vi "Get Children.vi"(8 "error in (no error)":errorcluster, 11 "Tag_LVOOP in":refnum<class "Tree Tag Class.lvclass">) -> (0 "error out":errorcluster, 1 "Child found?":bool, 2 "Children Tag Strings":string[](array[string]), 3 "Tag_LVOOP out":refnum<class "Tree Tag Class.lvclass">)   [LabVIEW 2012, in "Tree Tools.lvlib" / "Tree Tag Class.lvclass"]
uses:
  Tree Tag Class.lvclass
  Tree Tag Class.lvclass/Tree Tag Class.ctl
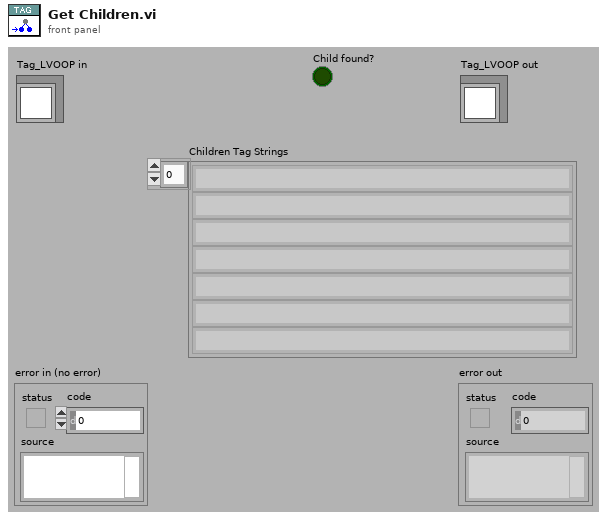
[diagram p1: front panel]
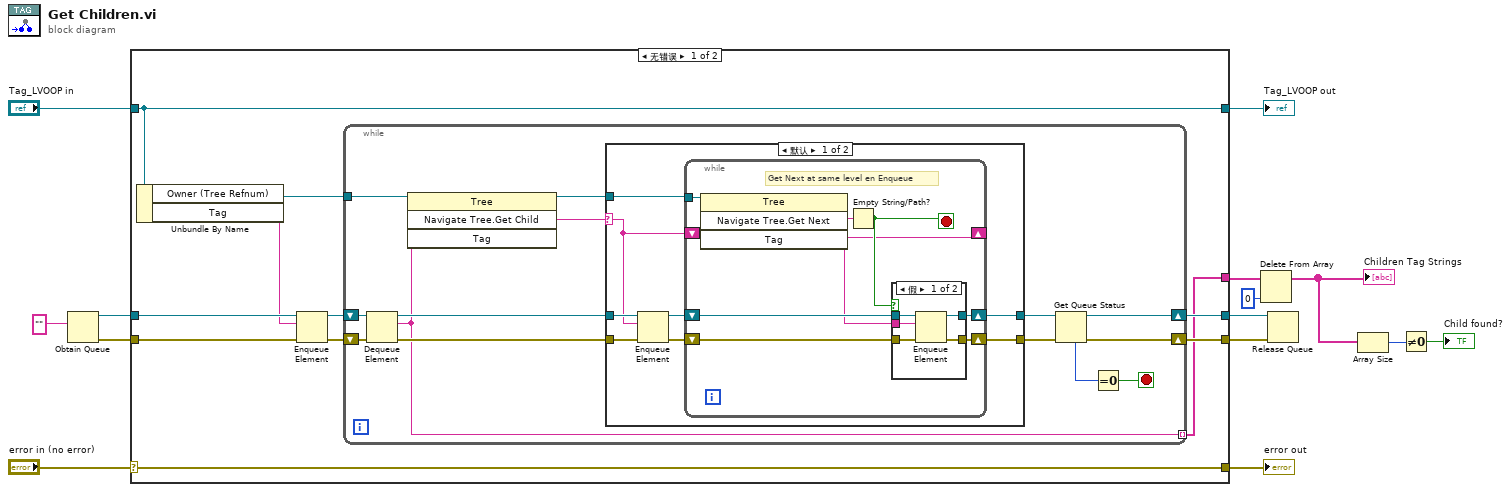
[diagram p0: block diagram]
diagram:
  n1 = Obtain Queue(element data type="") -> (queue out=w9:refnum<queue>, error out=w7:errorcluster)  [unwired: 3 in, 2 out]
  n2 = case shown="无错误" "error in (no error)" {
    selector: "error in (no error)" -> [w25 w68]
    tunnel: [w25 w68] -> w13
    tunnel: [w24 w67] -> w11
    tunnel: "Tag_LVOOP in" -> [w24 w67]
    tunnel: w9 -> [w20 w66]
    tunnel: [w22 w66] -> w8
    tunnel: w7 -> [w19 w65]
    tunnel: [w21 w65] -> w6
    tunnel: [w15 _] -> w5
    frame No Error {
      n3 = Unbundle By Name(w24) -> ("Owner (Tree Refnum)"=w23:refnum<vi>, "Tag"=w16:string)
      n4 = Enqueue Element(queue=w20, element=w16, error in (no error)=w19) -> (queue out=w18:refnum<queue>, error out=w17:errorcluster)  [unwired: 2 out]
      n5 = while {
        tunnel: w23 -> [w39]
        shift-right: [w31] -> w22
        shift-left: w18 -> [w37]
        shift-right: [w30] -> w21
        shift-left: w17 -> [w36]
        tunnel: [w27] -> w15 mode=indexing
        stop <- w28 stop-if-true
        n6 = Dequeue Element(queue=w37, error in (no error)=w36) -> (queue out=w35:refnum<queue>, element=w27:string, error out=w34:errorcluster)  [unwired: 2 out]
        n7 = invoke class="Tree" method="Navigate Tree.Get Child"(reference=w39, "Tag"=w27) -> (reference out=w38:refnum<vi>, "Navigate Tree:Get Child"=w26:string)  [unwired: 2 in, 2 out]
        n8 = case shown="默认" w26 {
          selector: w26 -> [w40 _]
          tunnel: w38 -> [w47 _]
          tunnel: w35 -> [w46 w64]
          tunnel: [w42 w64] -> w33
          tunnel: w34 -> [w45 w63]
          tunnel: [w41 w63] -> w32
          frame Default {
            n9 = Enqueue Element(queue=w46, element=w40, error in (no error)=w45) -> (queue out=w44:refnum<queue>, error out=w43:errorcluster)  [unwired: 2 out]
            n10 = while {
              tunnel: w47 -> [w55]
              shift-right: [w50] -> w41
              shift-left: w43 -> [w53]
              shift-right: [w51] -> w42
              shift-left: w44 -> [w54]
              shift-right: [w48] -> _
              shift-left: w40 -> [w49]
              stop <- w52 stop-if-true
              # "Get Next at same level en Enqueue"
              n11 = invoke class="Tree" method="Navigate Tree.Get Next"(reference=w55, "Tag"=w49) -> ("Navigate Tree:Get Next Item"=w48:string)  [unwired: 2 in, 3 out]
              n12 = Empty String/Path?(string/path=w48) -> (empty?=w52:bool)
              n13 = case shown="假" w52 {
                tunnel: w54 -> [w60 w62]
                tunnel: w53 -> [w59 w61]
                tunnel: w48 -> [w58 _]
                tunnel: [w57 w62] -> w51
                tunnel: [w56 w61] -> w50
                frame False {
                  n14 = Enqueue Element(queue=w60, element=w58, error in (no error)=w59) -> (queue out=w57:refnum<queue>, error out=w56:errorcluster)  [unwired: 2 out]
                }
                frame True {
                }
              }
            }
          }
          frame "" {
          }
        }
        n15 = Get Queue Status(queue=w33, error in (no error)=w32) -> (queue out=w31:refnum<queue>, error out=w30:errorcluster, # elements in queue=w29:i32)  [unwired: 6 out]
        n16 = Equal To 0?(x=w29) -> (x = 0?=w28:bool)
      }
    }
    frame Error {
    }
  }
  "error out" <- w13
  "Tag_LVOOP out" <- w11
  n17 = Delete From Array(array=w5, index=0) -> (array with subset deleted=w3:string[])  [unwired: 1 in, 1 out]
  "Children Tag Strings" <- w3
  n18 = Release Queue(queue=w8, error in (no error)=w6) -> ()  [unwired: 4 out]
  n19 = Array Size(array=w3) -> (size(s)=w2:i32)
  n20 = Not Equal To 0?(x=w2) -> (x != 0?=→"Child found?":bool)
